vi "convertExposureTime.vi"(8 "error in (no error)":errorcluster, 10 "time s":dbl, 11 "PixelflySettings in":refnum<class "PixelflySettings.lvclass">) -> (0 "error out":errorcluster, 2 "exposureTime":i32, 3 "PixelflySettings out":refnum<class "PixelflySettings.lvclass">)   [LabVIEW 2009, in "Tools.lvlib" / "Settings.lvlib" / "PixelflySettings.lvclass"]
uses:
  PixelflySettings.lvclass
  PixelflySettings.lvclass/PixelflySettings.ctl
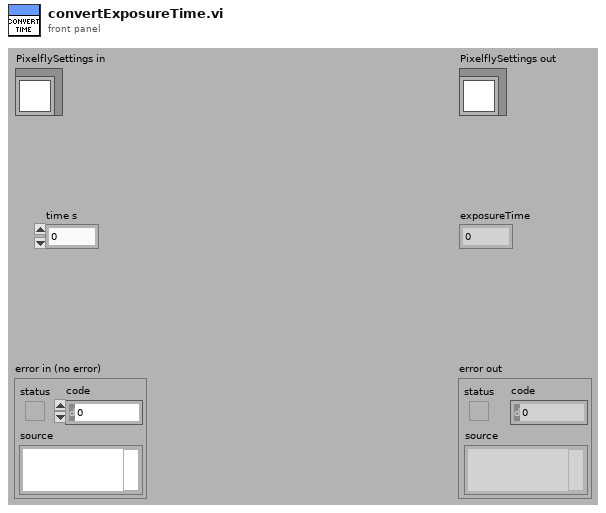
[diagram p1: front panel]
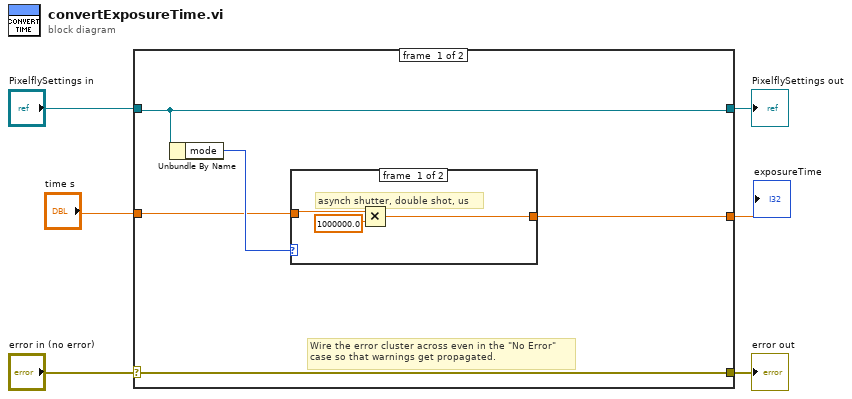
[diagram p0: block diagram]
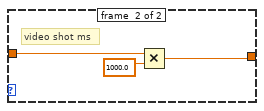
[diagram p2: hidden frame]
diagram:
  n1 = case shown="No Error" "error in (no error)" {
    selector: "error in (no error)" -> [w11 w19]
    tunnel: [w11 w19] -> w5
    tunnel: [w10 w18] -> w3
    tunnel: "PixelflySettings in" -> [w10 w18]
    tunnel: [w8 _] -> w2
    tunnel: "time s" -> [w7 _]
    frame #0 {
      # "Wire the error cluster across even in the \"No Error\"\ncase so that warnings get propagated."
      n2 = Unbundle By Name(w10) -> ("mode"=w9:u16)
      n3 = case shown="0, 1, Default" w9 {
        tunnel: w7 -> [w13 w17]
        tunnel: [w12 w16] -> w8
        frame #0 {
          # "asynch shutter, double shot, us"
          n4 = Multiply(x=w13, y=1000000.0) -> (x*y=w12:dbl)
        }
        frame #1 {
          # "video shot ms"
          n5 = Multiply(x=w17, y=1000.0) -> (x*y=w16:dbl)
        }
      }
    }
    frame #1 {
    }
  }
  "error out" <- w5
  "PixelflySettings out" <- w3
  "exposureTime" <- w2
